vi "interfaz.vi"() -> ()   [LabVIEW 2013]
uses:
  <vilib>/MakerHub/LINX/Public/Peripherals/Analog/Analog Read 1 Chan.vi
  <vilib>/MakerHub/LINX/Public/Peripherals/Analog/Analog Read N Chans.vi
  <vilib>/MakerHub/LINX/Private/Local IO/LinxAnalogRead.vi
  <vilib>/MakerHub/LINX/Public/Utilities/Check Channel.vi
  <vilib>/MakerHub/LINX/Public/Utilities/Open Serial.vi
  <vilib>/Utility/file.llb/Write To Spreadsheet File (DBL).vi
  <vilib>/MakerHub/LINX/Private/Utilties/Generate Error.vi
  <vilib>/Instr/_visa.llb/VISA Configure Serial Port (Instr).vi
  <vilib>/MakerHub/LINX/LMH-LINX.lvlib
panel:
  out "error out 2":errorcluster
  in  "Tab Control":T1(tab)=enum."Main"
  in  "Lap counter enable":bool=TRUE
  in  "Serial Port":refnum<visa-resource-name>="COM3"
  in  "Treshold":dbl(slide)=1.5656565656565655 scale=0.0..5.0
  out "Pass":bool
  out "Sensor 1":dbl
  out "Sensor 2":dbl
  out "Loop Rate (Hz)":u32=4294967295
  in  "file path (dialog if empty)":path=path "C:/Users/Pepe/Desktop/spiderLogs.csv"
  out "error out":errorcluster
  in  "Enable Termination\nChar (T)":bool
  in  "VISA resource name":refnum<visa-resource-name>="COM4"
  in  "button k":bool
  in  "Fan base":u16=280 max=999 step=1
  in  "button j":bool
  in  "Fan max":u16=300 max=999 step=1
  out "Bluetooth ready":bool=TRUE
  in  "button h":bool
  in  "button g":bool
  in  "button f":bool
  in  "button e":bool
  in  "button d":bool
  in  "button c":bool
  in  "button b":bool
  in  "button a":bool
  out "Arduino ready":bool
  out "Best time":dbl
  out "Previous time":dbl
  in  "Kd straight":u16=800 max=999 step=1
  in  "Kp straight":u16=9 max=999 step=1
  in  "Kd curve":u16=900 max=999 step=1
  in  "Kp curve":u16=14 max=999 step=1
  in  "Max speed straight":u8=100
  in  "Base speed straight":u8=100
  in  "Max speed curve":u8=100
  in  "Base speed curve":u8=100
  out "Laps":dbl
  out "Started":bool
  out "Enabled":bool=TRUE
  out "Time":dbl
  in  "Enable logging":bool
  in  "Run":bool=TRUE
  out "Line":dbl(knob)=-4.775461657315418 scale=-10.0..10.0
  in  "Diagnostics enable":bool
  out "Sensors":bool[](array[boolean])=[TRUE, TRUE, TRUE, TRUE, TRUE, TRUE, TRUE, TRUE, TRUE, TRUE, TRUE, TRUE, TRUE, TRUE, TRUE, TRUE, TRUE, TRUE]
  in  "stop":bool
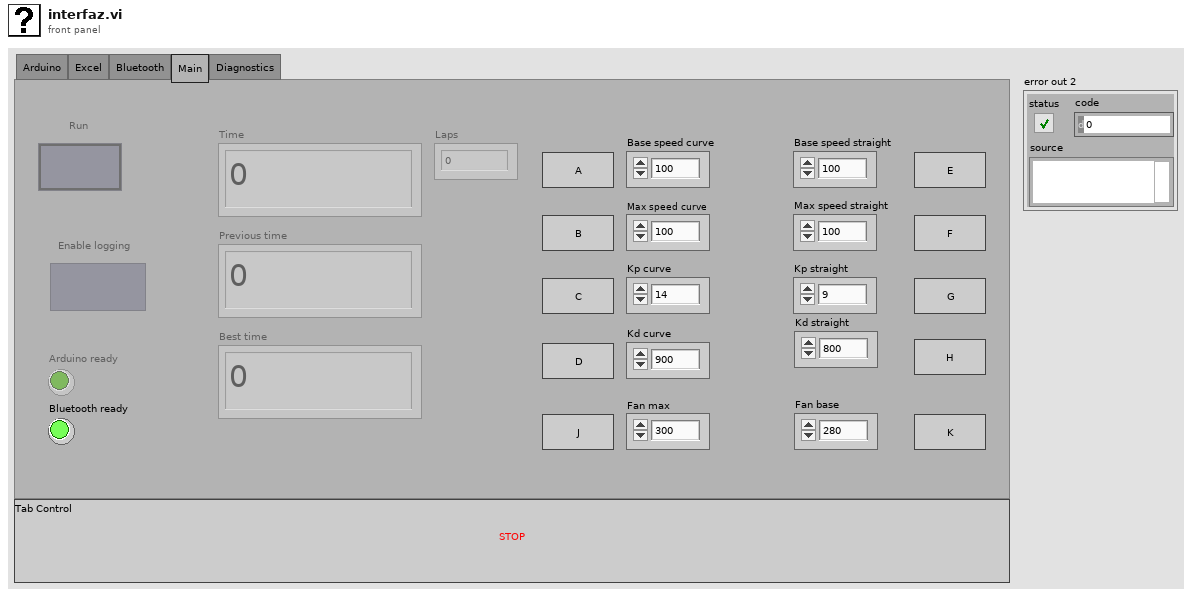
[diagram p1: front panel]
types:
  T1 = enum32{"Arduino", "Excel", "Bluetooth", "Main", "Diagnostics"}
  T2 = enum8{"Enabled", "Disabled", "Disabled and Grayed Out"}
  T3 = typedef "LMH-LINX.lvlib/LINX Ref.ctl" = cluster{"IO":T4, "Interface":T5, "LINX Device Config":T6}
  T4 = typedef "LMH-LINX.lvlib/Platform.ctl" = enum16{"Remote", "Local"}
  T5 = typedef "LMH-LINX.lvlib/Interface.ctl" = enum16{"Serial", "TCP"}
  T6 = typedef "LMH-LINX.lvlib/Device.lvlib/LINX Device Config.ctl" = cluster{"Interface":T5, "COM Port":refnum<visa-resource-name>, "TCP Configuration":T7, "Device Family":u8, "Device ID":u8, "Device Name":string, "TCP Ref":refnum<k5>, "Channels":T8}
  T7 = typedef "LMH-LINX.lvlib/Device.lvlib/TCP Config.ctl" = cluster{"IP Address":string, "Port":u16}
  T8 = typedef "LMH-LINX.lvlib/Channels.ctl" = cluster{"DI":u8[], "DO":u8[], "AI":u8[], "AO":u8[], "PWM":u8[], "QE":u8[], "UART":u8[], "I2C 2":u8[], "SPI":u8[], "CAN":u8[], "Servo":u8[], "AI Ref (V)":dbl, "AI Resolution (Bits)":u8, "AO Ref (V)":dbl, "AO Resolution (Bits)":u8}
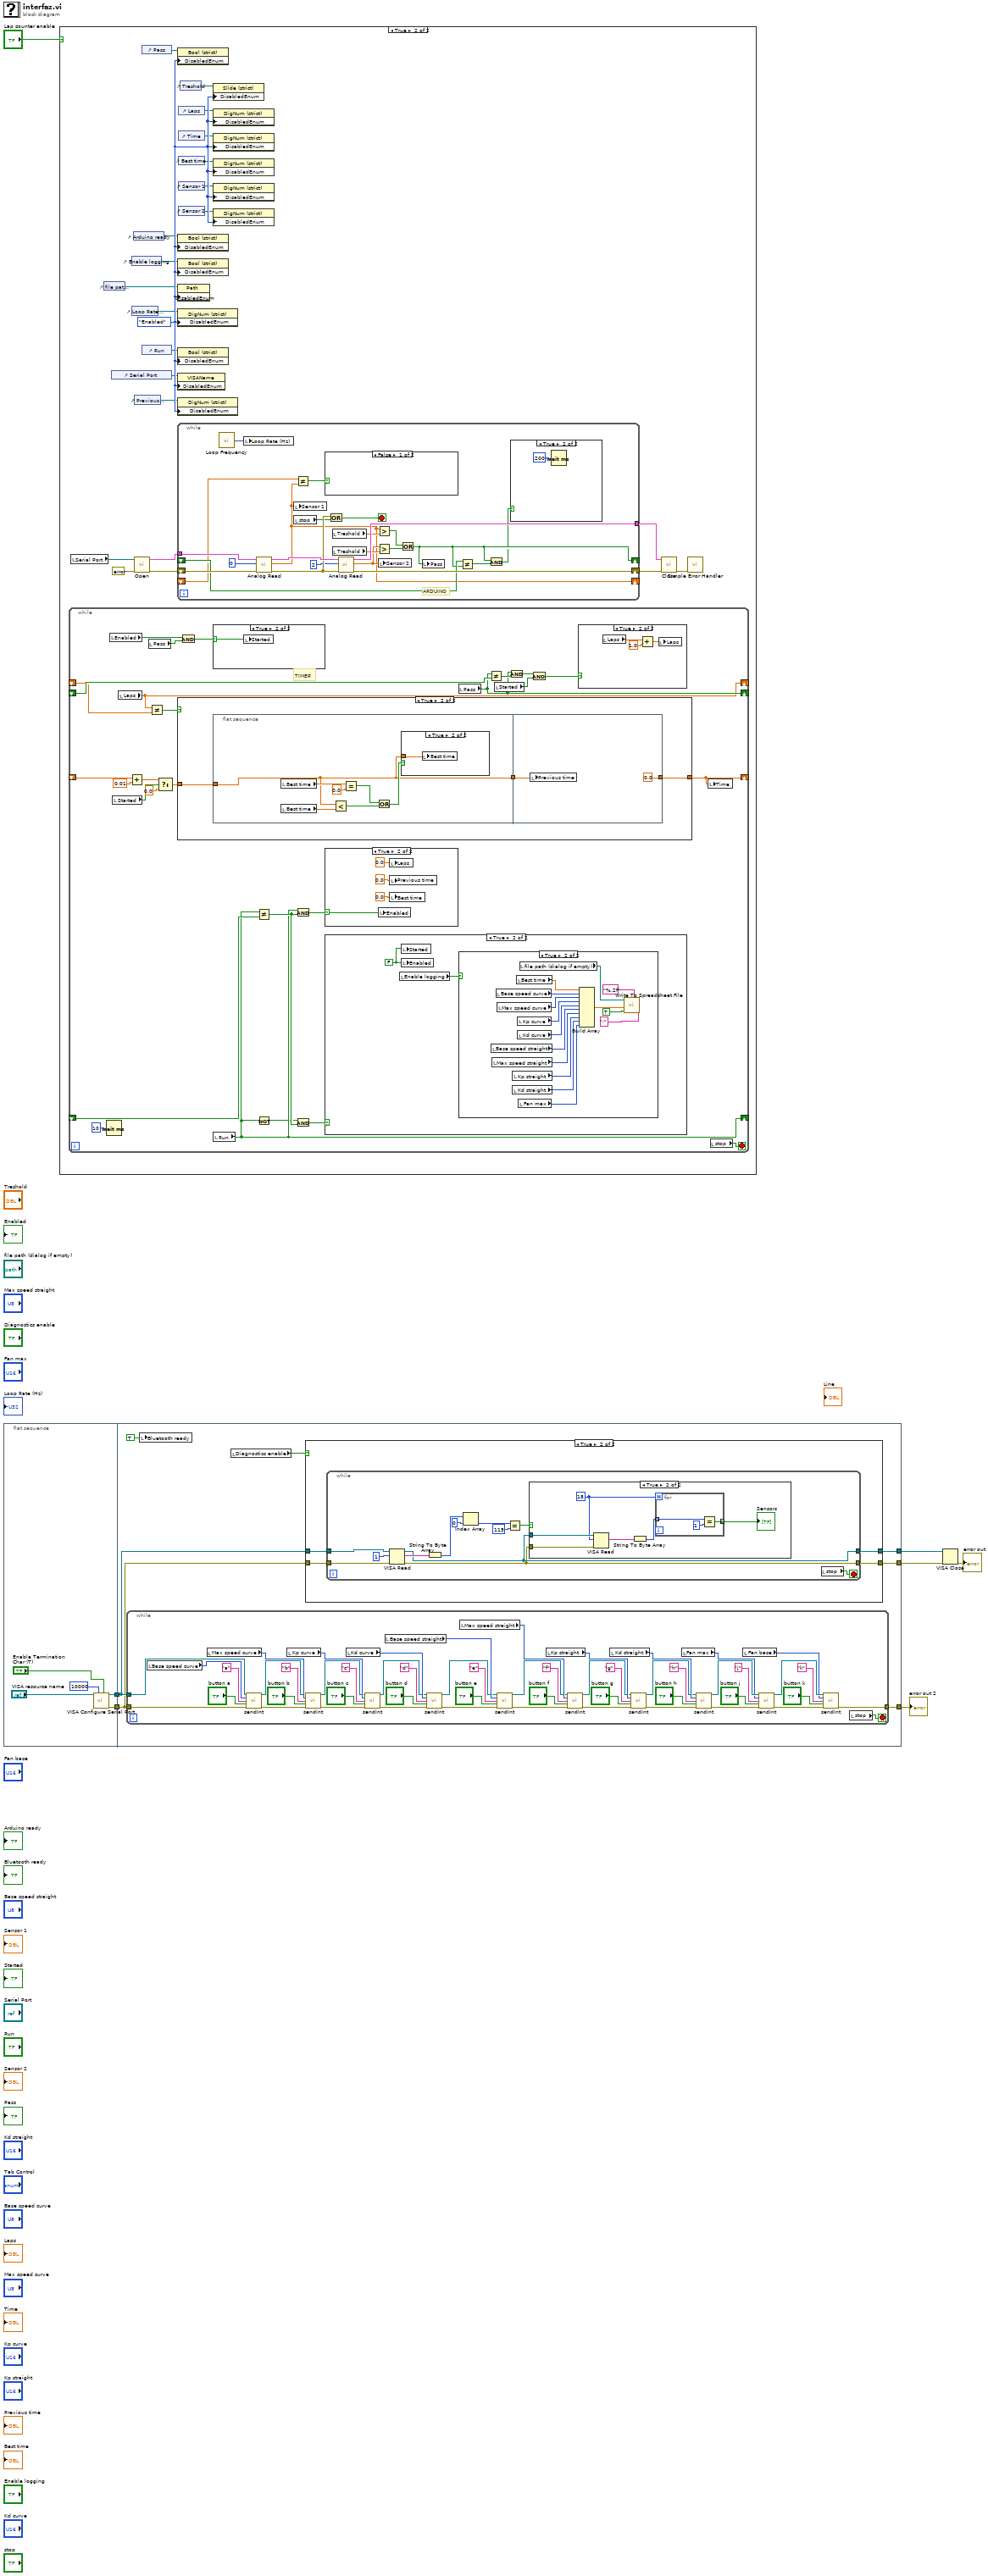
[diagram p0: block diagram]
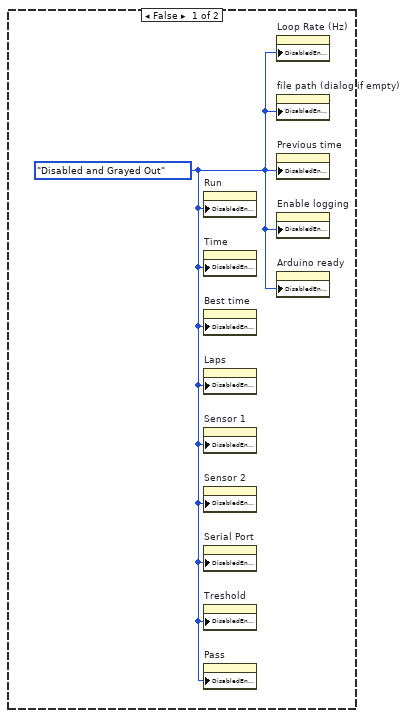
[diagram p4: hidden frame]
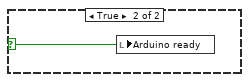
[diagram p12: hidden frame]
diagram:
  n1 = flat-sequence {
    tunnel: [w9] -> w6
    tunnel: [w8] -> w5
    tunnel: w6 -> [w18]
    tunnel: w5 -> [w17]
    tunnel: [w15] -> w3
    tunnel: [w14] -> w2
    tunnel: [w13] -> w1
    frame #0 {
      n2 = call-poly "VISA Configure Serial Port"("VISA resource name"="VISA resource name", "timeout (10sec)"=u32 10000, "Enable Termination\nChar (T)"="Enable Termination\nChar (T)") -> ("VISA resource name out"=w9:refnum<visa-resource-name>, "error out"=w8:errorcluster)  [unwired: 11 in]
    }
    frame #1 {
      n3 = while {
        tunnel: w18 -> [w60]
        tunnel: w17 -> [w59]
        tunnel: [w50] -> w13
        stop <- w58 stop-if-true
        n4 = local read "Base speed curve"() -> (w91:u8)
        n5 = local read "Max speed curve"() -> (w92:u8)
        n6 = call "sendInt.vi"("VISA resource name"=w60, "number"=w91, "letter"="a", "sender"="button a", "error in (no error)"=w59) -> ("VISA resource name out"=w82:refnum<visa-resource-name>, "error out"=w81:errorcluster)  [unwired: 9 in]
        n7 = local read "Kp curve"() -> (w93:u16)
        n8 = call "sendInt.vi"("VISA resource name"=w82, "number"=w92, "letter"="b", "sender"="button b", "error in (no error)"=w81) -> ("VISA resource name out"=w62:refnum<visa-resource-name>, "error out"=w67:errorcluster)  [unwired: 9 in]
        n9 = local read "Kd curve"() -> (w94:u16)
        n10 = call "sendInt.vi"("VISA resource name"=w62, "number"=w93, "letter"="c", "sender"="button c", "error in (no error)"=w67) -> ("VISA resource name out"=w63:refnum<visa-resource-name>, "error out"=w68:errorcluster)  [unwired: 9 in]
        n11 = local read "Base speed straight"() -> (w95:u8)
        n12 = call "sendInt.vi"("VISA resource name"=w63, "number"=w94, "letter"="d", "sender"="button d", "error in (no error)"=w68) -> ("VISA resource name out"=w64:refnum<visa-resource-name>, "error out"=w69:errorcluster)  [unwired: 9 in]
        n13 = local read "Max speed straight"() -> (w96:u8)
        n14 = call "sendInt.vi"("VISA resource name"=w64, "number"=w95, "letter"="e", "sender"="button e", "error in (no error)"=w69) -> ("VISA resource name out"=w65:refnum<visa-resource-name>, "error out"=w70:errorcluster)  [unwired: 9 in]
        n15 = local read "Kp straight"() -> (w97:u16)
        n16 = call "sendInt.vi"("VISA resource name"=w65, "number"=w96, "letter"="f", "sender"="button f", "error in (no error)"=w70) -> ("VISA resource name out"=w66:refnum<visa-resource-name>, "error out"=w71:errorcluster)  [unwired: 9 in]
        n17 = local read "Kd straight"() -> (w98:u16)
        n18 = call "sendInt.vi"("VISA resource name"=w66, "number"=w97, "letter"="g", "sender"="button g", "error in (no error)"=w71) -> ("VISA resource name out"=w79:refnum<visa-resource-name>, "error out"=w72:errorcluster)  [unwired: 9 in]
        n19 = local read "Fan max"() -> (w55:u16)
        n20 = call "sendInt.vi"("VISA resource name"=w79, "number"=w98, "letter"="h", "sender"="button h", "error in (no error)"=w72) -> ("VISA resource name out"=w57:refnum<visa-resource-name>, "error out"=w56:errorcluster)  [unwired: 9 in]
        n21 = local read "Fan base"() -> (w48:u16)
        n22 = call "sendInt.vi"("VISA resource name"=w57, "number"=w55, "letter"="j", "sender"="button j", "error in (no error)"=w56) -> ("VISA resource name out"=w52:refnum<visa-resource-name>, "error out"=w51:errorcluster)  [unwired: 9 in]
        n23 = call "sendInt.vi"("VISA resource name"=w52, "number"=w48, "letter"="k", "sender"="button k", "error in (no error)"=w51) -> ("error out"=w50:errorcluster)  [unwired: 9 in, 1 out]
        n24 = local read "stop"() -> (w58:bool)
      }
      n25 = local write "Bluetooth ready"(TRUE) -> ()
      n26 = local read "Diagnostics enable"() -> (w16:bool)
      n27 = case shown="True" w16 {
        tunnel: w18 -> [w21 w25]
        tunnel: w17 -> [w20 w24]
        tunnel: [w21 w23] -> w15
        tunnel: [w20 w22] -> w14
        frame False {
        }
        frame True {
          n28 = while {
            tunnel: w25 -> [w37]
            tunnel: w24 -> [w36]
            tunnel: [w26] -> w22
            tunnel: [w27] -> w23
            stop <- w29 stop-if-true
            n29 = VISA Read(VISA resource name=w37, byte count=u32 1, error in (no error)=w36) -> (VISA resource name out=w27:refnum<visa-resource-name>, read buffer=w34:string, error out=w26:errorcluster)  [unwired: 1 out]
            n30 = String To Byte Array(string=w34) -> (unsigned byte array=w33:u8[])
            n31 = Index Array(array=w33, index=0) -> (element=w28:u8)
            n32 = Equal?(x=w28, y=u8 115) -> (x = y?=w30:bool)
            n33 = case shown="True" w30 {
              tunnel: w27 -> [_ w43]
              tunnel: w26 -> [_ w42]
              frame False {
              }
              frame True {
                w41 = 18
                n34 = VISA Read(VISA resource name=w43, byte count=w41, error in (no error)=w42) -> (read buffer=w40:string)  [unwired: 3 out]
                n35 = String To Byte Array(string=w40) -> (unsigned byte array=w39:u8[])
                n36 = for {
                  N: w41 -> [_]
                  tunnel: w39 -> [w46] mode=indexing
                  tunnel: [w44] -> w38 mode=indexing
                  n37 = Equal?(x=w46, y=u8 1) -> (x = y?=w44:bool)
                }
                "Sensors" <- w38
              }
            }
            n38 = local read "stop"() -> (w29:bool)
          }
        }
      }
    }
  }
  n39 = case shown="True" "Lap counter enable" {
    frame False {
      w99 = T2."Disabled and Grayed Out" ("Disabled")
      n40 = property on="Run" class="Bool (strict)"("DisabledEnum"=w99) -> ()  [unwired: 2 in, 2 out]
      n41 = property on="Time" class="DigNum (strict)"("DisabledEnum"=w99) -> ()  [unwired: 2 in, 2 out]
      n42 = property on="Best time" class="DigNum (strict)"("DisabledEnum"=w99) -> ()  [unwired: 2 in, 2 out]
      n43 = property on="Laps" class="DigNum (strict)"("DisabledEnum"=w99) -> ()  [unwired: 2 in, 2 out]
      n44 = property on="Sensor 1" class="DigNum (strict)"("DisabledEnum"=w99) -> ()  [unwired: 2 in, 2 out]
      n45 = property on="Sensor 2" class="DigNum (strict)"("DisabledEnum"=w99) -> ()  [unwired: 2 in, 2 out]
      n46 = property on="Serial Port" class="VISAName"("DisabledEnum"=w99) -> ()  [unwired: 2 in, 2 out]
      n47 = property on="Treshold" class="Slide (strict)"("DisabledEnum"=w99) -> ()  [unwired: 2 in, 2 out]
      n48 = property on="Pass" class="Bool (strict)"("DisabledEnum"=w99) -> ()  [unwired: 2 in, 2 out]
      n49 = property on="Loop Rate (Hz)" class="DigNum (strict)"("DisabledEnum"=w99) -> ()  [unwired: 2 in, 2 out]
      n50 = property on="file path (dialog if empty)" class="Path"("DisabledEnum"=w99) -> ()  [unwired: 2 in, 2 out]
      n51 = property on="Previous time" class="DigNum (strict)"("DisabledEnum"=w99) -> ()  [unwired: 2 in, 2 out]
      n52 = property on="Enable logging" class="Bool (strict)"("DisabledEnum"=w99) -> ()  [unwired: 2 in, 2 out]
      n53 = property on="Arduino ready" class="Bool (strict)"("DisabledEnum"=w99) -> ()  [unwired: 2 in, 2 out]
    }
    frame True {
      w115 = T2."Enabled" ("Disabled")
      n54 = while {
        shift-right: [w128] -> _
        shift-left: _ -> [w148]
        shift-right: [w125] -> _
        shift-left: _ -> [w145]
        shift-right: [w135] -> _
        shift-left: _ -> [w137]
        shift-right: [w130] -> _
        shift-left: _ -> [w129]
        stop <- w133 stop-if-true
        # "TIMER"
        n55 = Wait (ms)(milliseconds to wait=u32 10) -> ()  [unwired: 1 out]
        n56 = local read "Enabled"() -> (w143:bool)
        n57 = local read "Started"() -> (w139:bool)
        n58 = local read "Laps"() -> (w130:dbl)
        n59 = Add(x=w148, y=0.01) -> (x+y=w141:dbl)
        n60 = local read "Pass"() -> (w142:bool)
        n61 = Not Equal?(x=w130, y=w129) -> (x != y?=w122:bool)
        n62 = Select(t=w141, s=w139, f=0.0) -> (s? t:f=w127:dbl)
        n63 = case shown="True" w122 {
          tunnel: [w166 w167] -> w128
          tunnel: w127 -> [w166 w169]
          frame False {
          }
          frame True {
            n64 = flat-sequence {
              tunnel: w169 -> [w171]
              tunnel: [w171] -> w168
              tunnel: w168 -> [w179]
              tunnel: [0.0] -> w167
              frame #0 {
                n65 = local read "Best time"() -> (w174:dbl)
                n66 = local read "Best time"() -> (w170:dbl)
                n67 = Less?(x=w171, y=w170) -> (x < y?=w173:bool)
                n68 = Equal?(x=w174, y=0.0) -> (x = y?=w175:bool)
                n69 = Or(x=w175, y=w173) -> (x .or. y?=w172:bool)
                n70 = case shown="True" w172 {
                  tunnel: w171 -> [_ w177]
                  frame False {
                  }
                  frame True {
                    n71 = local write "Best time"(w177) -> ()
                  }
                }
              }
              frame #1 {
                n72 = local write "Previous time"(w179) -> ()
              }
            }
          }
        }
        n73 = And(x=w143, y=w142) -> (x .and. y?=w140:bool)
        n74 = case shown="True" w140 {
          selector: w140 -> [_ w183]
          frame False {
          }
          frame True {
            n75 = local write "Started"(w183) -> ()
          }
        }
        n76 = local read "Run"() -> (w125:bool)
        n77 = Not Equal?(x=w125, y=w145) -> (x != y?=w126:bool)
        n78 = Not(x=w125) -> (.not. x?=w124:bool)
        n79 = And(x=w125, y=w126) -> (x .and. y?=w144:bool)
        n80 = And(x=w124, y=w126) -> (x .and. y?=w123:bool)
        n81 = case shown="True" w144 {
          selector: w144 -> [_ w187]
          frame False {
          }
          frame True {
            n82 = local write "Enabled"(w187) -> ()
            n83 = local write "Laps"(0.0 ("Laps")) -> ()
            n84 = local write "Previous time"(0.0 ("Previous time")) -> ()
            n85 = local write "Best time"(0.0 ("Best time")) -> ()
          }
        }
        n86 = case shown="True" w123 {
          frame False {
          }
          frame True {
            w150 = FALSE ("Enabled")
            n87 = local read "Enable logging"() -> (w149:bool)
            n88 = local write "Started"(w150) -> ()
            n89 = local write "Enabled"(w150) -> ()
            n90 = case shown="True" w149 {
              frame False {
              }
              frame True {
                n91 = local read "Base speed straight"() -> (w157:u8)
                n92 = local read "Max speed straight"() -> (w156:u8)
                n93 = local read "Base speed curve"() -> (w161:u8)
                n94 = local read "Max speed curve"() -> (w160:u8)
                n95 = local read "Kp straight"() -> (w155:u16)
                n96 = local read "Kd straight"() -> (w154:u16)
                n97 = local read "Best time"() -> (w162:dbl)
                n98 = local read "Kp curve"() -> (w159:u16)
                n99 = local read "Kd curve"() -> (w158:u16)
                n100 = local read "Fan max"() -> (w151:u16)
                n101 = local read "file path (dialog if empty)"() -> (w152:path)
                n102 = Build Array(w162, w161, w160, w159, w158, w157, w156, w155, w154, w151) -> (w153:dbl[])
                n103 = call-poly <vilib>:"Write To Spreadsheet File.vi"("delimiter (\\t)"=";" ("delimiter (\\t)"), "format (%.3f)"="%.2f", "append to file? (new file:F)"=TRUE, "1D data"=w153, "file path (dialog if empty)"=w152) -> ()  [unwired: 3 in, 1 out]
              }
            }
          }
        }
        n104 = local read "Pass"() -> (w135:bool)
        n105 = Not Equal?(x=w135, y=w137) -> (x != y?=w136:bool)
        n106 = local read "Started"() -> (w132:bool)
        n107 = And(x=w135, y=w136) -> (x .and. y?=w134:bool)
        n108 = And(x=w134, y=w132) -> (x .and. y?=w131:bool)
        n109 = case shown="True" w131 {
          frame False {
          }
          frame True {
            n110 = local read "Laps"() -> (w180:dbl)
            n111 = Add(x=w180, y=1.0) -> (x+y=w181:dbl)
            n112 = local write "Laps"(w181) -> ()
          }
        }
        n113 = local write "Time"(w128) -> ()
        n114 = local read "stop"() -> (w133:bool)
      }
      n115 = local read "Serial Port"() -> (w104:refnum<visa-resource-name>)
      n116 = control-ref of="file path (dialog if empty)"() -> (w113:refnum<vi>)
      n117 = control-ref of="Serial Port"() -> (w101:refnum<vi>)
      n118 = control-ref of="Enable logging"() -> (w105:refnum<vi>)
      n119 = control-ref of="Loop Rate (Hz)"() -> (w103:refnum<vi>)
      n120 = control-ref of="Arduino ready"() -> (w112:refnum<vi>)
      n121 = control-ref of="Previous time"() -> (w107:refnum<vi>)
      n122 = call-poly <vilib>:"Open.vi"("Error In"=errorcluster {"status"=FALSE, "code"=0, "source"=""}, "Serial Port"=w104) -> ("Error Out"=w119:errorcluster, "LINX Resource"=w120:T3)  [unwired: 7 in, 1 out]
      n123 = control-ref of="Pass"() -> (w111:refnum<vi>)
      n124 = control-ref of="Run"() -> (w109:refnum<vi>)
      n125 = property on="Property Node" class="Bool (strict)"(reference=w111, "DisabledEnum"=w115) -> ()  [unwired: 1 in, 2 out]
      n126 = property on="Property Node" class="Bool (strict)"(reference=w112, "DisabledEnum"=w115) -> ()  [unwired: 1 in, 2 out]
      n127 = property on="Property Node" class="Bool (strict)"(reference=w105, "DisabledEnum"=w115) -> ()  [unwired: 1 in, 2 out]
      n128 = property on="Property Node" class="Path"(reference=w113, "DisabledEnum"=w115) -> ()  [unwired: 1 in, 2 out]
      n129 = property on="Property Node" class="DigNum (strict)"(reference=w103, "DisabledEnum"=w115) -> ()  [unwired: 1 in, 2 out]
      n130 = property on="Property Node" class="Bool (strict)"(reference=w109, "DisabledEnum"=w115) -> ()  [unwired: 1 in, 2 out]
      n131 = property on="Property Node" class="VISAName"(reference=w101, "DisabledEnum"=w115) -> ()  [unwired: 1 in, 2 out]
      n132 = property on="Property Node" class="DigNum (strict)"(reference=w107, "DisabledEnum"=w115) -> ()  [unwired: 1 in, 2 out]
      n133 = while {
        tunnel: w120 -> [w210]
        tunnel: [w204] -> w117
        shift-right: [w203] -> w116
        shift-left: w119 -> [w209]
        shift-right: [w194] -> _
        shift-left: _ -> [w196]
        shift-right: [w189] -> _
        shift-left: _ -> [w190]
        stop <- w207 stop-if-true
        # "ARDUINO"
        n134 = call <vilib>:"Loop Frequency.vi"() -> ("Loop Rate (Hz)"=w191:u32)
        n135 = local write "Loop Rate (Hz)"(w191) -> ()
        n136 = call-poly <vilib>:"Analog Read.vi"("Error In"=w209, "Analog Channel"=u8 0, "LINX Resource"=w210) -> ("Error Out"=w205:errorcluster, "Voltage"=w189:dbl, "LINX Resource"=w206:T3)  [unwired: 5 in, 1 out]
        n137 = local write "Sensor 1"(w189) -> ()
        n138 = local read "stop"() -> (w201:bool)
        n139 = Not Equal?(x=w190, y=w189) -> (x != y?=w188:bool)
        n140 = case shown="False" w188 {
          selector: w188 -> [_ w211]
          frame False {
          }
          frame True {
            n141 = local write "Arduino ready"(w211) -> ()
          }
        }
        n142 = Or(x=w205, y=w201) -> (x .or. y?=w207:bool)
        n143 = local read "Treshold"() -> (w200:dbl)
        n144 = local read "Treshold"() -> (w197:dbl)
        n145 = call-poly <vilib>:"Analog Read.vi"("Error In"=w205, "Analog Channel"=u8 2, "LINX Resource"=w206) -> ("Error Out"=w203:errorcluster, "Voltage"=w192:dbl, "LINX Resource"=w204:T3)  [unwired: 5 in, 1 out]
        n146 = Greater?(x=w189, y=w200) -> (0:w199:bool)
        n147 = Greater?(x=w192, y=w197) -> (0:w198:bool)
        n148 = local write "Sensor 2"(w192) -> ()
        n149 = Or(x=w199, y=w198) -> (x .or. y?=w194:bool)
        n150 = local write "Pass"(w194) -> ()
        n151 = Not Equal?(x=w196, y=w194) -> (x != y?=w195:bool)
        n152 = And(x=w194, y=w195) -> (x .and. y?=w193:bool)
        n153 = case shown="True" w193 {
          frame False {
          }
          frame True {
            n154 = Wait (ms)(milliseconds to wait=u32 200) -> ()  [unwired: 1 out]
          }
        }
      }
      n155 = control-ref of="Laps"() -> (w110:refnum<vi>)
      n156 = control-ref of="Time"() -> (w108:refnum<vi>)
      n157 = control-ref of="Best time"() -> (w106:refnum<vi>)
      n158 = control-ref of="Sensor 1"() -> (w102:refnum<vi>)
      n159 = control-ref of="Sensor 2"() -> (w100:refnum<vi>)
      n160 = control-ref of="Treshold"() -> (w114:refnum<vi>)
      n161 = property on="Property Node" class="Slide (strict)"(reference=w114, "DisabledEnum"=w115) -> ()  [unwired: 1 in, 2 out]
      n162 = property on="Property Node" class="DigNum (strict)"(reference=w110, "DisabledEnum"=w115) -> ()  [unwired: 1 in, 2 out]
      n163 = property on="Property Node" class="DigNum (strict)"(reference=w108, "DisabledEnum"=w115) -> ()  [unwired: 1 in, 2 out]
      n164 = property on="Property Node" class="DigNum (strict)"(reference=w106, "DisabledEnum"=w115) -> ()  [unwired: 1 in, 2 out]
      n165 = property on="Property Node" class="DigNum (strict)"(reference=w102, "DisabledEnum"=w115) -> ()  [unwired: 1 in, 2 out]
      n166 = property on="Property Node" class="DigNum (strict)"(reference=w100, "DisabledEnum"=w115) -> ()  [unwired: 1 in, 2 out]
      n167 = call <vilib>:"Close.vi"("Error In"=w116, "LINX Resource"=w117) -> ("Error Out"=w118:errorcluster)  [unwired: 9 in]
      n168 = call <vilib>:"Simple Error Handler.vi"("error in (no error)"=w118) -> ()  [unwired: 4 in, 5 out]
    }
  }
  n169 = VISA Close(VISA resource name=w3, error in (no error)=w2) -> (error out=→"error out":errorcluster)
  "error out 2" <- w1
